vi "DriveModuleControlLogic.vi"(8 "Pass_Through_Time":dbl=-1.0 format="%33.4f", 9 "Actual State":T1 {"Angle"."SIN" format="%13.4f"; "Angle"."COS" format="%13.4f"; "Angle"."VALUE" format="%13.4f"}, 10 "Desired State":T1={"Speed"=0.0, "Angle"={"VALUE"=0.0, "COS"=1.0, "SIN"=0.0}} {"Angle"."SIN" format="%13.4f"; "Angle"."COS" format="%13.4f"; "Angle"."VALUE" format="%13.4f"}, 11 "ModualNamePrefix":i32) -> (2 "SpinMotorDmd":dbl, 3 "TravelMotorDmd":dbl)   [LabVIEW 2023]
uses:
  <vilib>/Rock Robotics/WPI/ThirdParty/JAS_Junk/TrajLib/TypeDef/SWERVE_DRIVE_MODULE_STATE.ctl
  <vilib>/Rock Robotics/WPI/ThirdParty/JAS_Junk/TrajLib/TypeDef/ROTATION2D.ctl
  <vilib>/Rock Robotics/WPI/ThirdParty/JAS_Junk/TrajLib/Rotation2d_Minus.vi
  <vilib>/Rock Robotics/WPI/ThirdParty/JAS_Junk/TrajLib/Rotation2d_GetRadians.vi
  <vilib>/Rock Robotics/WPI/ThirdParty/JAS_Junk/TrajLib/SwerveModuleState_New.vi
  <vilib>/Rock Robotics/WPI/ThirdParty/JAS_Junk/TrajLib/Rotation2d_RotateBy.vi
  <vilib>/Rock Robotics/WPI/ThirdParty/JAS_Junk/TrajLib/Rotation2d_CreateAngle.vi
  <vilib>/Rock Robotics/WPI/ThirdParty/JAS_Junk/TrajLib/SimpleMotorFF_Calculate.vi
  <vilib>/Rock Robotics/WPI/ThirdParty/JAS_Junk/TrajLib/PIDController_AtSetpoint.vi
  <vilib>/Rock Robotics/WPI/ThirdParty/JAS_Junk/TrajLib/PIDController_SetPIDF.vi
  <vilib>/Rock Robotics/WPI/ThirdParty/JAS_Junk/TrajLib/PIDController_SetDerivativeFilter.vi
  <vilib>/Rock Robotics/WPI/ThirdParty/JAS_Junk/TrajLib/PIDController_SetIntegratorRange.vi
  <vilib>/Rock Robotics/WPI/ThirdParty/JAS_Junk/TrajLib/PIDController_SetTolerancePandV.vi
  <vilib>/Rock Robotics/WPI/ThirdParty/JAS_Junk/TrajLib/PIDController_DisableContinousInput.vi
  <vilib>/Rock Robotics/WPI/ThirdParty/JAS_Junk/TrajLib/PIDController_EnableContinousInput.vi
  <vilib>/Rock Robotics/WPI/ThirdParty/JAS_Junk/TrajLib/PIDController_Reset.vi
  <vilib>/Rock Robotics/WPI/ThirdParty/JAS_Junk/TrajLib/PIDController_New.vi
  <vilib>/Rock Robotics/WPI/ThirdParty/JAS_Junk/TrajLib/PIDController_SetOutputLimits.vi
  <vilib>/Rock Robotics/WPI/ThirdParty/JAS_Junk/TrajLib/VI/PIDController_SetIntegratorZone.vi
  <vilib>/Rock Robotics/WPI/ThirdParty/JAS_Junk/TrajLib/SlewRateLimiter_New.vi
  <vilib>/Rock Robotics/WPI/ThirdParty/JAS_Junk/TrajLib/SlewRateLimiter_Reset.vi
  <vilib>/Rock Robotics/WPI/ThirdParty/JAS_Junk/TrajLib/SlewRateLimiter_Calculate.vi
  <vilib>/Rock Robotics/WPI/ThirdParty/JAS_Junk/TrajLib/SlewRateLimiter_SetRate.vi
  <vilib>/Rock Robotics/WPI/ThirdParty/JAS_Junk/TrajLib/VI/Util_GetTime_U32.vi
  <vilib>/Rock Robotics/WPI/ThirdParty/JAS_Junk/TrajLib/Rotation2d_UnaryMinus.vi
  <vilib>/Rock Robotics/WPI/ThirdParty/JAS_Junk/TrajLib/Rotation2d_CreateXY.vi
  <vilib>/Rock Robotics/WPI/ThirdParty/JAS_Junk/TrajLib/PIDController_NewPeriod.vi
  <vilib>/Rock Robotics/WPI/ThirdParty/JAS_Junk/TrajLib/Util_CalcDist.vi
  <vilib>/Rock Robotics/SystemInterfaces/NetworkCommunication/NetComm_UsageReport_report.vi
  Robot Global Data.vi
  DriveGlobal.vi
  <vilib>/Rock Robotics/SystemInterfaces/Utilities/FPGA_UtilitiesRead LocalTime.vi
  <vilib>/Rock Robotics/WPI/ThirdParty/JAS_Junk/TrajLib/VI/Util_GetTime_U64.vi
  <vilib>/Rock Robotics/WPI/ThirdParty/JAS_Junk/TrajLib/Globals/Util_LibraryGlobals.vi
  <vilib>/Rock Robotics/WPI/ThirdParty/JAS_Junk/TrajLib/PIDController_AdvCalculate_FF_Sp_Pv.vi
  <vilib>/Rock Robotics/WPI/ThirdParty/JAS_Junk/TrajLib/Trajectory_Library.lvlib
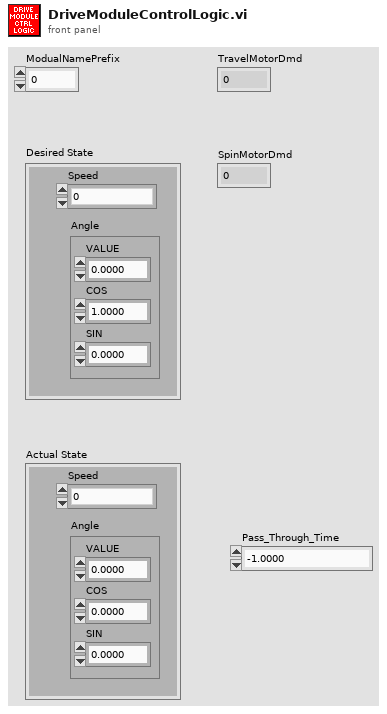
[diagram p1: front panel]
types:
  T1 = typedef "Trajectory_Library.lvlib/SWERVE_DRIVE_MODULE_STATE.ctl" = cluster{"Speed":dbl, "Angle":T2}
  T2 = typedef "Trajectory_Library.lvlib/ROTATION2D.ctl" = cluster{"VALUE":dbl, "COS":dbl, "SIN":dbl}
  T3 = typedef "Trajectory_Library.lvlib/SIMPLE_MOTOR_FF.ctl" = cluster{"Ks":dbl, "Kv":dbl, "Ka":dbl, "KnInv":dbl}
  T4 = typedef "Trajectory_Library.lvlib/PID_ADV_LIMITS.ctl" = cluster{"MaxInput":dbl, "MinInput":dbl, "Continuous":bool, "MaxOutput":dbl, "MinOutput":dbl}
  T5 = typedef "Trajectory_Library.lvlib/PID_ADV_TUNING.ctl" = cluster{"Kf":dbl, "Kp":dbl, "Ki":dbl, "Kd":dbl, "MaximumIntegral":dbl, "MinimumIntegral":dbl, "Filter Derivative":bool, "IntegralZone":dbl}
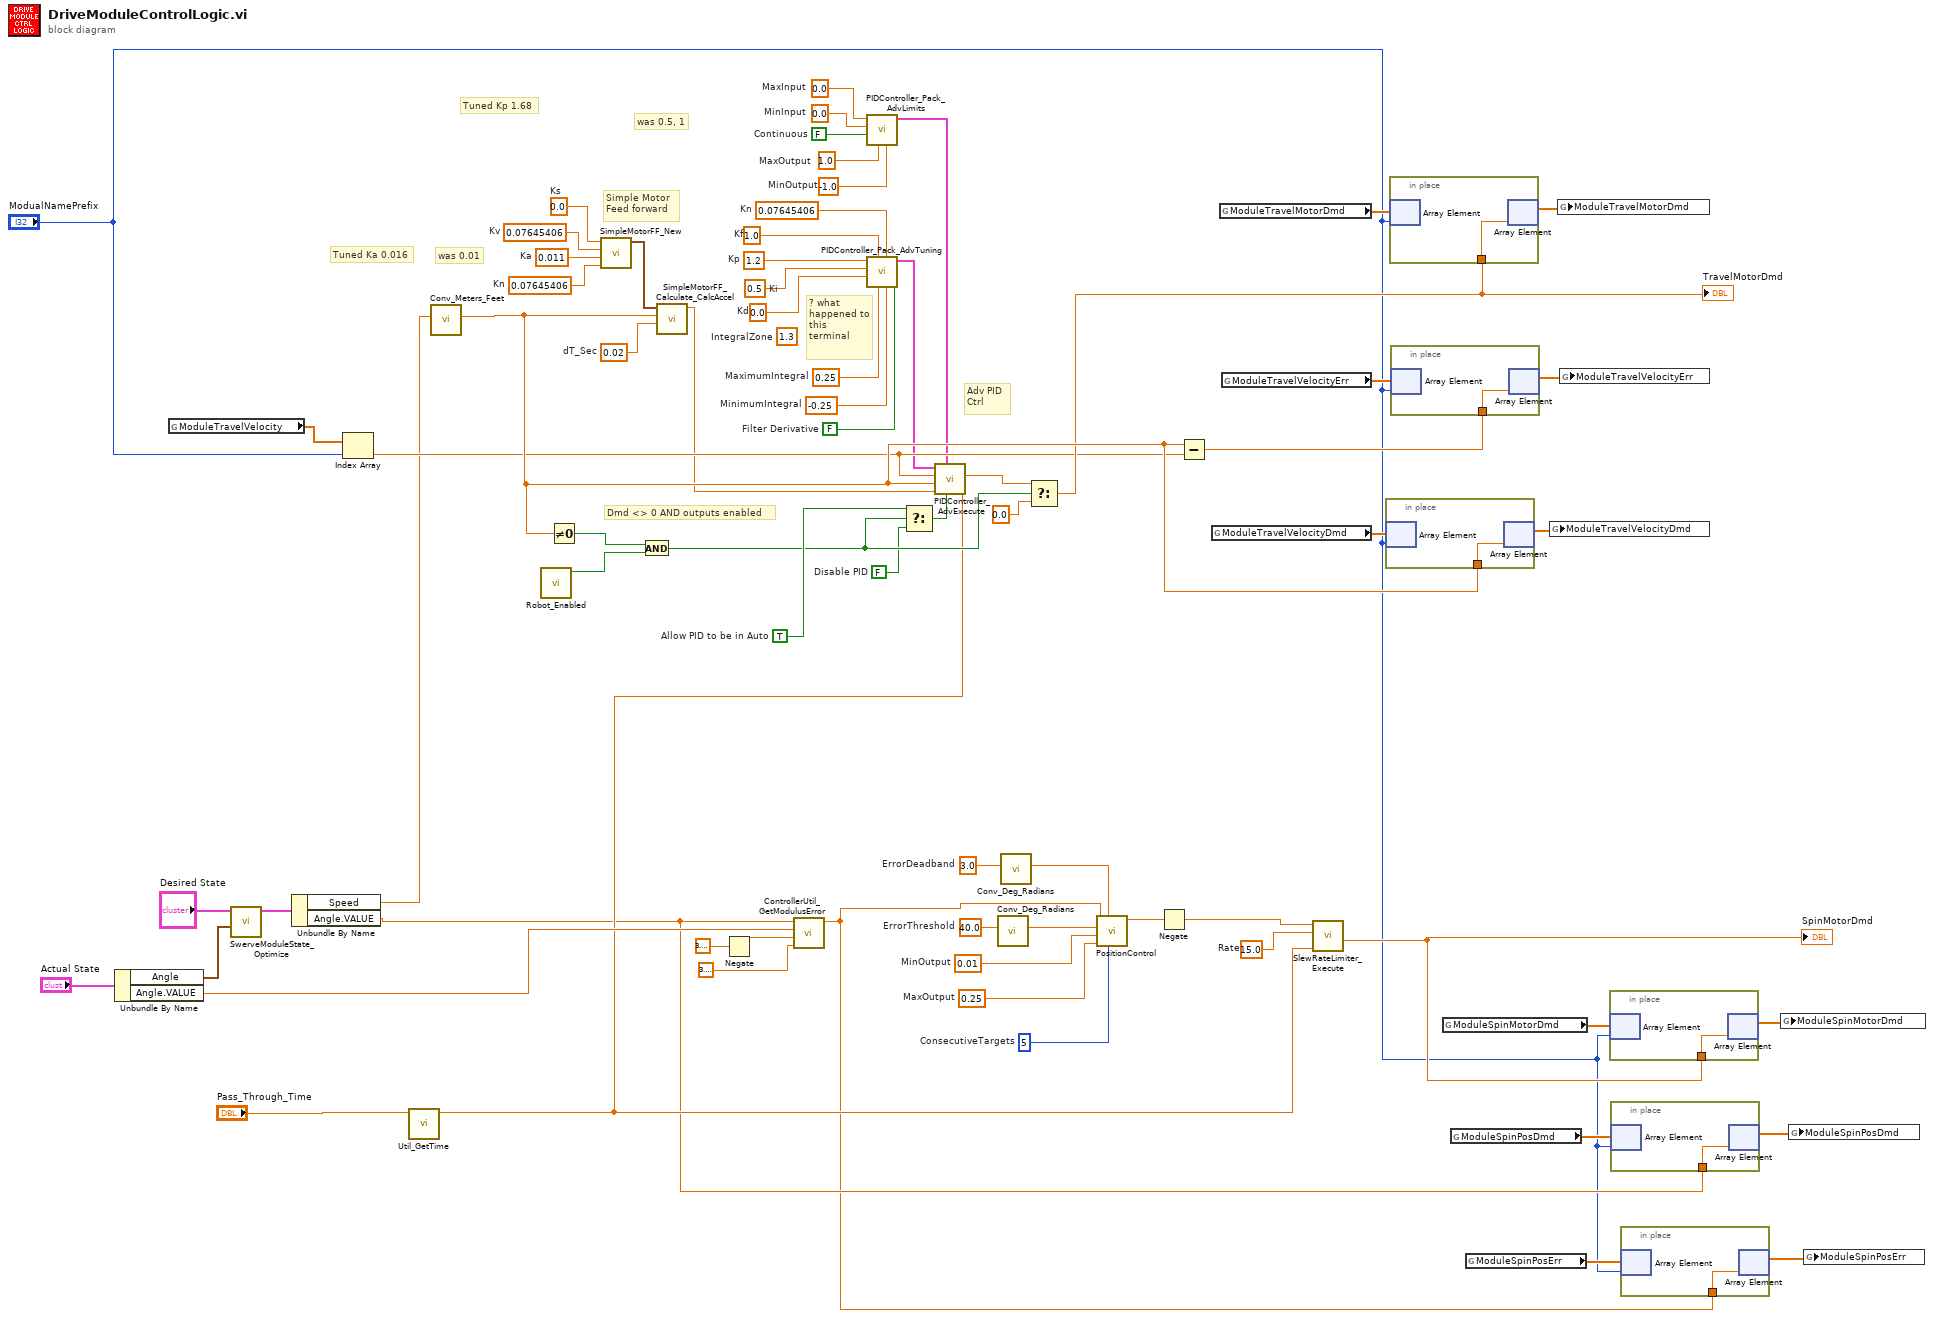
[diagram p0: block diagram]
diagram:
  (unwired) 1.3  # IntegralZone
  w59 = 15.0  # Rate
  w58 = TRUE  # Allow PID to be in Auto
  w56 = FALSE  # Disable PID
  w50 = 0.07645406  # Kn
  w34 = 1.2  # Kp
  w35 = 0.5  # Ki
  w36 = 0.0  # Kd
  w37 = 1.0  # Kf
  w38 = 0.25  # MaximumIntegral
  w39 = -0.25  # MinimumIntegral
  w40 = FALSE  # Filter Derivative
  w42 = 0.0  # MinInput
  w43 = FALSE  # Continuous
  w44 = 1.0  # MaxOutput
  w41 = -1.0  # MinOutput
  w45 = 0.0  # MaxInput
  w28 = 0.07645406  # Kn
  w29 = 0.02  # dT_Sec
  w31 = 0.0  # Ks
  w32 = 0.07645406  # Kv
  w33 = 0.011  # Ka
  w20 = 5  # ConsecutiveTargets
  w21 = 0.25  # MaxOutput
  w19 = 0.01  # MinOutput
  w24 = 40.0  # ErrorThreshold
  w22 = 3.0  # ErrorDeadband
  # "Tuned Kp 1.68"
  # "Tuned Ka 0.016"
  # "was 0.01"
  # "? what happened to this terminal"
  # "was 0.5, 1"
  # "Dmd <> 0 AND outputs enabled"
  # "Adv PID\nCtrl"
  # "Simple Motor\nFeed forward"
  n1 = Unbundle By Name("Actual State") -> ("Angle"=w13:T2, "Angle.VALUE"=w16:dbl)
  n2 = global read "DriveGlobal.vi" "ModuleTravelVelocity"() -> (w49:dbl[])
  n3 = call <vilib>:"SwerveModuleState_Optimize.vi"("CurrentAngle"=w13, "Desired State"="Desired State") -> ("out SWERVE_DRIVE_MODULE_STATE"=w15:T1)  [unwired: 9 in]
  n4 = Unbundle By Name(w15) -> ("Speed"=w27:dbl, "Angle.VALUE"=w5:dbl)
  n5 = Index Array(array=w49, index="ModualNamePrefix") -> (element=w51:dbl)
  n6 = call <vilib>:"Util_GetTime.vi"("Pass_Through_Time"="Pass_Through_Time") -> ("FPGA_Time_Seconds"=w10:dbl)  [unwired: 8 in, 2 out]
  n7 = call <vilib>:"Conv_Meters_Feet.vi"("Meters"=w27) -> ("Feet"=w69:dbl)  [unwired: 10 in]
  n8 = call "Robot_Enabled.vi"() -> ("Robot Enabled"=w8:bool)  [unwired: 11 in]
  n9 = Not Equal To 0?(x=w69) -> (x != 0?=w54:bool)
  n10 = call <vilib>:"SimpleMotorFF_New.vi"("Kn"=w28, "Ka"=w33, "Kv"=w32, "Ks"=w31) -> ("SIMPLE_MOTOR_FF"=w30:T3)  [unwired: 7 in]
  n11 = And(x=w54, y=w8) -> (x .and. y?=w57:bool)
  n12 = call <vilib>:"SimpleMotorFF_Calculate_CalcAccel.vi"("dT_Sec"=w29, "VelSp"=w69, "SIMPLE_MOTOR_FF"=w30) -> ("FeedForward"=w48:dbl)  [unwired: 8 in]
  n13 = Negate(x=3.141592653589793) -> (-x=w14:dbl)
  n14 = call <vilib>:"ControllerUtil_GetModulusError.vi"("Maximum_Input"=3.141592653589793, "Minimum_Input"=w14, "Measurerment(PV)"=w16, "Reference(SP)"=w5) -> ("Error"=w1:dbl)  [unwired: 7 in]
  n15 = call <vilib>:"PIDController_Pack_AdvLimits.vi"("MinOutput"=w41, "MaxOutput"=w44, "Continuous"=w43, "MinInput"=w42, "MaxInput"=w45) -> ("Adv PID Limits"=w47:T4)  [unwired: 6 in]
  n16 = call <vilib>:"PIDController_Pack_AdvTuning.vi"("Filter Derivative"=w40, "MinimumIntegral"=w39, "Kn"=w50, "MaximumIntegral"=w38, "Kf"=w37, "Kd"=w36, "Ki"=w35, "Kp"=w34) -> ("Adv PID Tuning"=w46:T5)  [unwired: 3 in]
  n17 = Select(t=w58, s=w57, f=w56) -> (s? t:f=w55:bool)
  n18 = call <vilib>:"PIDController_AdvExecute.vi"("Time"=w10, "Auto"=w55, "Adv PID Limits"=w47, "FF-FeedForward"=w48, "SP-SetPoint"=w69, "PV-Measurement"=w51, "Adv PID Tuning"=w46) -> ("CO-ControlOutput"=w52:dbl)  [unwired: 2 in, 2 out]
  n19 = call <vilib>:"Conv_Deg_Radians.vi"("Degress"=w24) -> ("Radians"=w25:dbl)  [unwired: 10 in]
  n20 = call <vilib>:"Conv_Deg_Radians.vi"("Degress"=w22) -> ("Radians"=w23:dbl)  [unwired: 10 in]
  n21 = Select(t=w52, s=w57, f=0.0 ("t")) -> (s? t:f=w63:dbl)
  "TravelMotorDmd" <- w63
  n22 = call "PositionControl.vi"("ConsecutiveTargets"=w20, "ErrorDeadband"=w23, "MaxOutput"=w21, "MinOutput"=w19, "ErrorThreshold"=w25, "Error"=w1) -> ("OutputValue"=w26:dbl)  [unwired: 3 in, 2 out]
  n23 = Negate(x=w26) -> (-x=w60:dbl)
  n24 = Subtract(x=w69, y=w51) -> (x-y=w66:dbl)
  n25 = global read "DriveGlobal.vi" "ModuleTravelVelocityDmd"() -> (w67:dbl[])
  n26 = global read "DriveGlobal.vi" "ModuleTravelMotorDmd"() -> (w61:dbl[])
  n27 = global read "DriveGlobal.vi" "ModuleTravelVelocityErr"() -> (w64:dbl[])
  n28 = call <vilib>:"SlewRateLimiter_Execute.vi"("Time"=w10, "PositiveRate"=w59, "Input"=w60) -> ("Output"=w72:dbl)  [unwired: 7 in, 1 out]
  "SpinMotorDmd" <- w72
  n29 = in-place {
    in-place-border: w69 -> [w73]
    n30 = in-place-array #1(w67, "ModualNamePrefix") -> ()  [unwired: 1 out]
    n31 = in-place-array #1(w73) -> (w68:dbl[])  [unwired: 1 out]
  }
  n32 = in-place {
    in-place-border: w63 -> [w74]
    n33 = in-place-array #2(w61, "ModualNamePrefix") -> ()  [unwired: 1 out]
    n34 = in-place-array #2(w74) -> (w62:dbl[])  [unwired: 1 out]
  }
  n35 = in-place {
    in-place-border: w66 -> [w75]
    n36 = in-place-array #3(w64, "ModualNamePrefix") -> ()  [unwired: 1 out]
    n37 = in-place-array #3(w75) -> (w65:dbl[])  [unwired: 1 out]
  }
  n38 = global read "DriveGlobal.vi" "ModuleSpinMotorDmd"() -> (w70:dbl[])
  n39 = global read "DriveGlobal.vi" "ModuleSpinPosDmd"() -> (w6:dbl[])
  n40 = global read "DriveGlobal.vi" "ModuleSpinPosErr"() -> (w3:dbl[])
  n41 = global write "DriveGlobal.vi" "ModuleTravelVelocityDmd"(w68) -> ()
  n42 = global write "DriveGlobal.vi" "ModuleTravelMotorDmd"(w62) -> ()
  n43 = global write "DriveGlobal.vi" "ModuleTravelVelocityErr"(w65) -> ()
  n44 = in-place {
    in-place-border: w72 -> [w76]
    n45 = in-place-array #4(w70, "ModualNamePrefix") -> ()  [unwired: 1 out]
    n46 = in-place-array #4(w76) -> (w71:dbl[])  [unwired: 1 out]
  }
  n47 = in-place {
    in-place-border: w5 -> [w77]
    n48 = in-place-array #5(w6, "ModualNamePrefix") -> ()  [unwired: 1 out]
    n49 = in-place-array #5(w77) -> (w7:dbl[])  [unwired: 1 out]
  }
  n50 = in-place {
    in-place-border: w1 -> [w78]
    n51 = in-place-array #6(w3, "ModualNamePrefix") -> ()  [unwired: 1 out]
    n52 = in-place-array #6(w78) -> (w4:dbl[])  [unwired: 1 out]
  }
  n53 = global write "DriveGlobal.vi" "ModuleSpinMotorDmd"(w71) -> ()
  n54 = global write "DriveGlobal.vi" "ModuleSpinPosDmd"(w7) -> ()
  n55 = global write "DriveGlobal.vi" "ModuleSpinPosErr"(w4) -> ()
